vi "KE622x -- Get Current Range.vi"(0 "Resource In":refnum<visa-resource-name>, 1 "Check For SCPI Errors? (T)":bool=TRUE, 11 "error in (no error)":errorcluster) -> (4 "Resource Out (dupl)":refnum<visa-resource-name>, 8 "Current Range":T1, 15 "error out":errorcluster)   [LabVIEW 2013, in "Keithly user program.lvlib"]
doc: "Returns the state of auto-ranging and the selected range. Note that the selected range was selected by the instrument if auto-range is True, else it was previously specified by the user."
uses:
  Keithly user program.lvlib
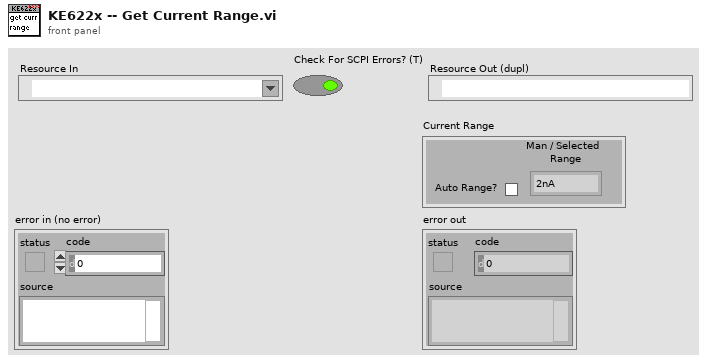
[diagram p1: front panel]
types:
  T1 = cluster{"Auto Range?":bool, "Man / Selected\n        Range":enum16{"2nA", "20nA", "200nA", "2uA", "20uA", "200uA", "2mA", "20mA", "100mA"}}
  T2 = enum16{"2nA", "20nA", "200nA", "2uA", "20uA", "200uA", "2mA", "20mA", "100mA"}
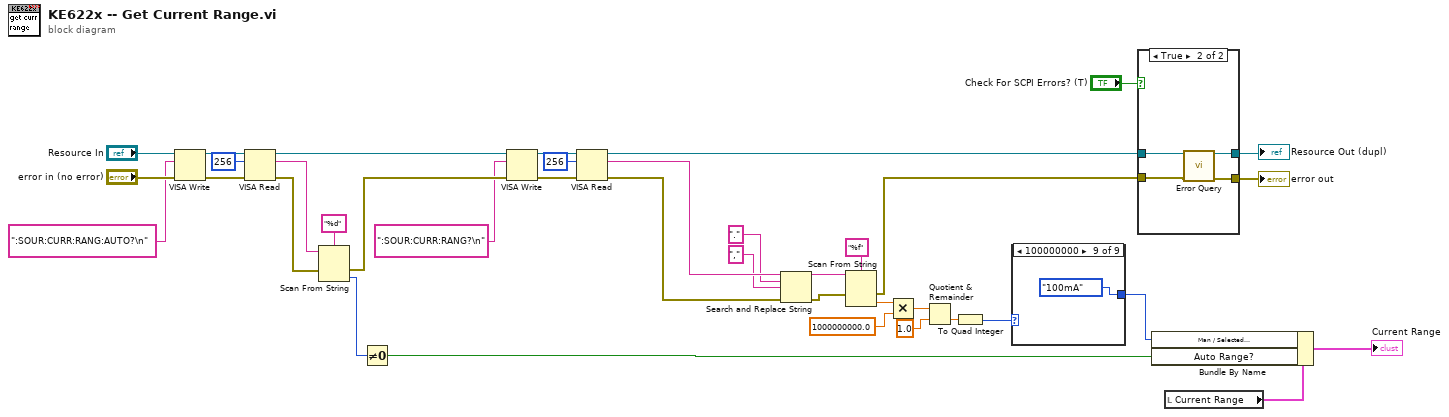
[diagram p0: block diagram]
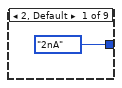
[diagram p2: hidden frame]
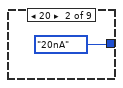
[diagram p3: hidden frame]
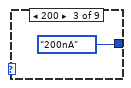
[diagram p4: hidden frame]
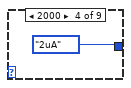
[diagram p5: hidden frame]
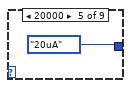
[diagram p6: hidden frame]
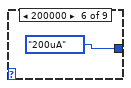
[diagram p7: hidden frame]
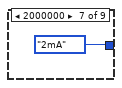
[diagram p8: hidden frame]
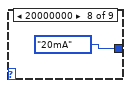
[diagram p9: hidden frame]
diagram:
  n1 = VISA Write(VISA resource name="Resource In", write buffer=":SOUR:CURR:RANG:AUTO?\n" ("format string"), error in (no error)="error in (no error)") -> (VISA resource name out=w32:refnum<visa-resource-name>, error out=w31:errorcluster)  [unwired: 1 out]
  n2 = VISA Read(VISA resource name=w32, byte count=u32 256, error in (no error)=w31) -> (VISA resource name out=w21:refnum<visa-resource-name>, read buffer=w27:string, error out=w29:errorcluster)  [unwired: 1 out]
  n3 = Scan From String(format string="%d", input string=w27, error in=w29) -> (error out=w22:errorcluster, output 1=w26:i32)  [unwired: 2 in, 2 out]
  n4 = Not Equal To 0?(x=w26) -> (x != 0?=w17:bool)
  n5 = VISA Write(VISA resource name=w21, write buffer=":SOUR:CURR:RANG?\n" ("format string"), error in (no error)=w22) -> (VISA resource name out=w25:refnum<visa-resource-name>, error out=w24:errorcluster)  [unwired: 1 out]
  n6 = VISA Read(VISA resource name=w25, byte count=u32 256, error in (no error)=w24) -> (VISA resource name out=w19:refnum<visa-resource-name>, read buffer=w5:string, error out=w4:errorcluster)  [unwired: 1 out]
  n7 = Search and Replace String(input string=w5, search string=".", replace string="," ("replace string (\"\")"), error in=w4) -> (result string=w6:string, error out=w3:errorcluster)  [unwired: 4 in, 2 out]
  n8 = Scan From String(format string="%f", input string=w6, error in=w3) -> (error out=w9:errorcluster, output 1=w15:dbl)  [unwired: 2 in, 2 out]
  n9 = Multiply(x=w15, y=1000000000.0) -> (x*y=w13:dbl)
  n10 = Quotient & Remainder(x=w13, y=1.0) -> (floor(x/y)=w11:dbl)  [unwired: 1 out]
  n11 = To Quad Integer(1:w11) -> (0:w10:i64)
  n12 = case shown="100000000" w10 {
    tunnel: [T2."2nA" ("Current Range") T2."20nA" ("Current Range") T2."200nA" ("Current Range") T2."2uA" ("Current Range") T2."20uA" ("Current Range") T2."200uA" ("Current Range") T2."2mA" ("Current Range") T2."20mA" ("Current Range") T2."100mA" ("Current Range")] -> w7
    frame 2, Default {
    }
    frame 20 {
    }
    frame 200 {
    }
    frame 2000 {
    }
    frame 20000 {
    }
    frame 200000 {
    }
    frame 2000000 {
    }
    frame 20000000 {
    }
    frame 100000000 {
    }
  }
  n13 = case shown="True" "Check For SCPI Errors? (T)" {
    tunnel: w19 -> [w49 w53]
    tunnel: w9 -> [w48 w50]
    tunnel: [w48 w51] -> w34
    tunnel: [w49 w52] -> w35
    frame False {
    }
    frame True {
      n14 = call "Error Query.vi"("VISA Resource In"=w53, "error in (no error)"=w50) -> ("VISA Resource Out (dupl)"=w52:refnum<visa-resource-name>, "error out"=w51:errorcluster)  [unwired: 10 in, 2 out]
    }
  }
  "Resource Out (dupl)" <- w35
  "error out" <- w34
  n15 = local read "Current Range"() -> (w18:T1)
  n16 = Bundle By Name(cluster=w18, "Man / Selected\n        Range"=w7, "Auto Range?"=w17) -> (→"Current Range":T1)
